vi "Part 1.vi"() -> ()   [LabVIEW 2020]
uses:
  <vilib>/Utility/file.llb/Read Delimited Spreadsheet (string).vi
panel:
  out "Histogram Graph":cluster{i32[], i32[]}(graph)
  out "sum":i32
  out "Array":string[](array[string])
  out "Map":map{string, i32}(c390)
  out "sorted array":cluster{string, i32}[](array[cluster])
  in  "Path":path
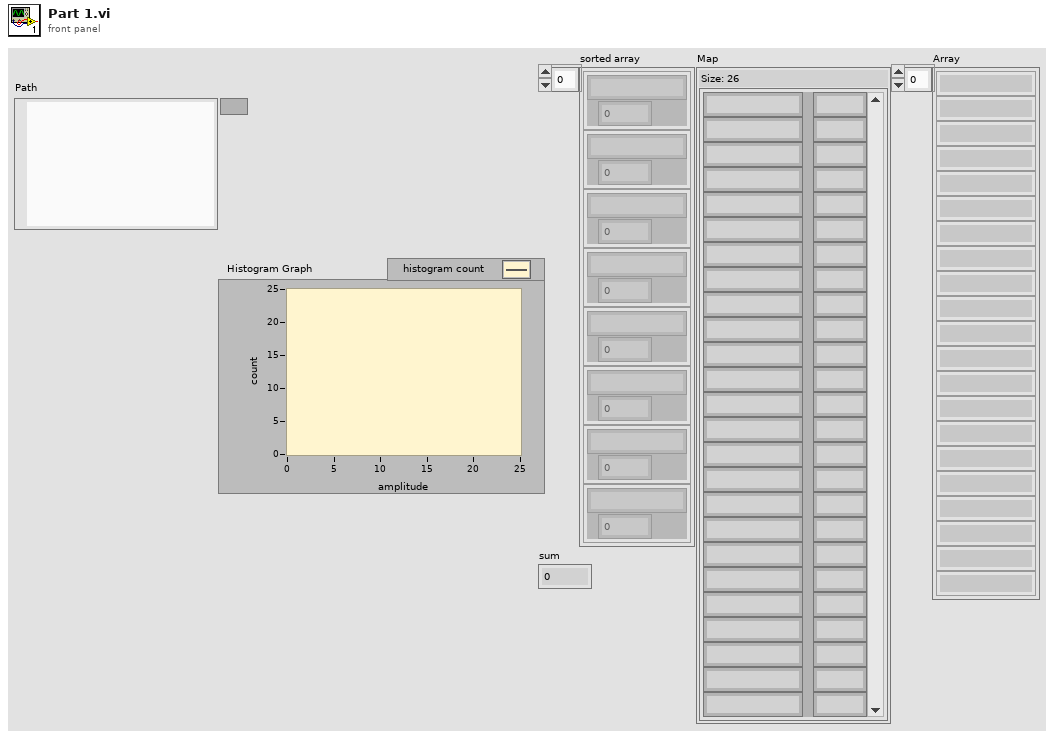
[diagram p1: front panel]
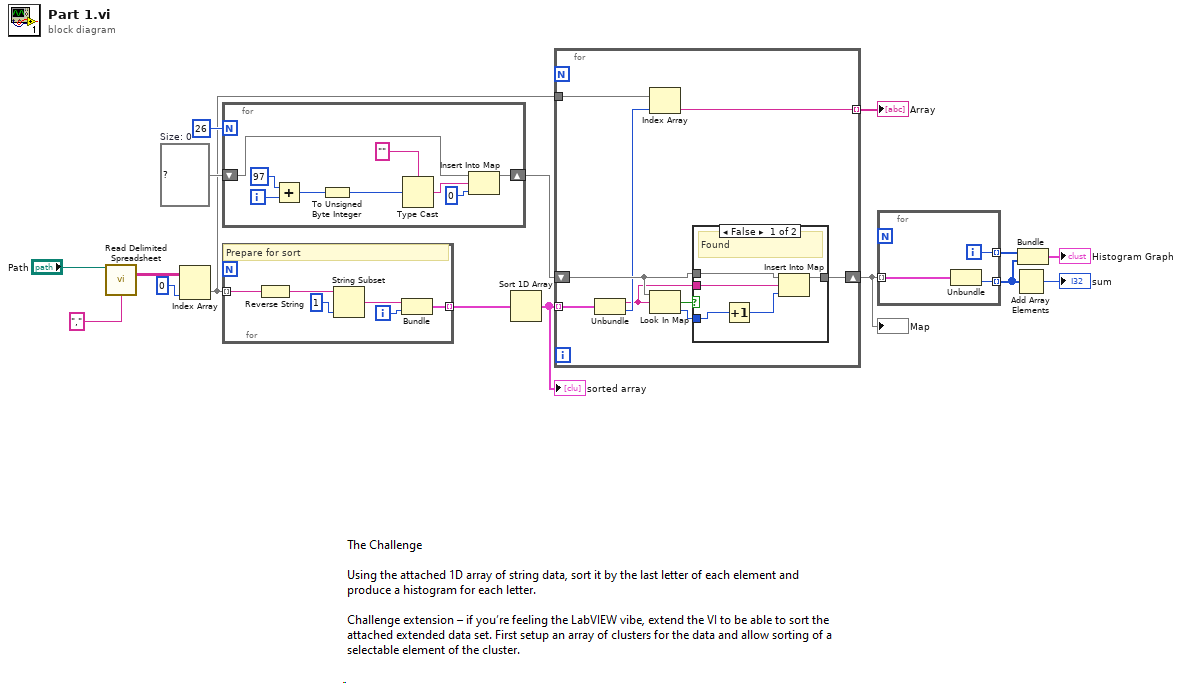
[diagram p0: block diagram]
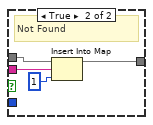
[diagram p2: hidden frame]
diagram:
  w11 = map{string, i32} {}  # Size: 0
  n1 = call-poly <vilib>:"Read Delimited Spreadsheet.vi"("file path (dialog if empty)"="Path", "delimiter (\\t)"="," ("delimiter (\\t)")) -> ("all rows"=w14:string[][])  [unwired: 8 in, 5 out]
  n2 = Index Array(array=w14, index (col)=0 ("disabled index (col)")) -> (element=w7:string[])  [unwired: 1 in]
  n3 = for {
    N: 26 -> [_]
    shift-right: [w20] -> w8
    shift-left: w11 -> [w21]
    i -> [w24]
    n4 = Add(x=97, y=w24) -> (x+y=w23:i32)
    n5 = To Unsigned Byte Integer(number=w23) -> (unsigned 8bit integer=w17:u8)
    n6 = Type Cast(type="", x=w17) -> (*(type *) &x=w19:string)
    n7 = Insert Into Map(map in=w21, key=w19, value=0) -> (map out=w20:map{string, i32})  [unwired: 2 out]
  }
  n8 = for {
    tunnel: w7 -> [w31] mode=indexing
    tunnel: [w26] -> w12 mode=indexing
    i -> [w27]
    # "Prepare for sort"
    n9 = Reverse String(1:w31) -> (0:w30:string)
    n10 = String Subset(string=w30, length (rest)=1 ("length (rest)")) -> (substring=w28:string)  [unwired: 1 in]
    n11 = Bundle(w28, w27) -> (w26:cluster{string, i32})  [unwired: 1 in]
  }
  n12 = Sort 1D Array(array=w12) -> (sorted array=w9:cluster{string, i32}[])
  "sorted array" <- w9
  n13 = for {
    tunnel: w9 -> [w40] mode=indexing
    shift-right: [w35] -> w5
    shift-left: w8 -> [w36]
    tunnel: w7 -> [w39]
    tunnel: [w38] -> w6 mode=indexing
    n14 = Unbundle(w40) -> (w33:string, w34:i32)
    n15 = Index Array(array=w39, index=w34) -> (element=w38:string)
    n16 = Look In Map(map=w36, key=w33) -> (key not found?=w37:bool, value=w32:i32)  [unwired: 1 in]
    n17 = case shown="False" w37 {
      tunnel: w36 -> [w45 w48]
      tunnel: [w44 w49] -> w35
      tunnel: w33 -> [w43 w47]
      tunnel: w32 -> [w42 _]
      frame False {
        # "Found"
        n18 = Increment(x=w42) -> (x+1=w41:i32)
        n19 = Insert Into Map(map in=w45, key=w43, value=w41) -> (map out=w44:map{string, i32})  [unwired: 2 out]
      }
      frame True {
        # "Not Found"
        n20 = Insert Into Map(map in=w48, key=w47, value=1) -> (map out=w49:map{string, i32})  [unwired: 2 out]
      }
    }
  }
  "Map" <- w5
  "Array" <- w6
  n21 = for {
    tunnel: w5 -> [w52] mode=indexing
    tunnel: [w51] -> w2 mode=indexing
    tunnel: [w50] -> w1 mode=indexing
    i -> [w50]
    n22 = Unbundle(w52) -> (w51:i32)  [unwired: 1 out]
  }
  n23 = Add Array Elements(numeric array=w2) -> (sum=→"sum":i32)
  n24 = Bundle(w1, w2) -> (→"Histogram Graph":cluster{i32[], i32[]})  [unwired: 1 in]
